vi "Choreo_SwerveSample_Unpack.vi"(9 "StartByte":i32, 11 "RawData":u8[](array[numeric])) -> (1 "NextByte":i32, 3 "ChoreoSwerveSample":T1)   [LabVIEW 2019, in "ChoreoLib.lvlib"]
doc: "Unpack a binary byte stream into a Swerve Trajectory Sample.\n\nInputs:\n -- RawData - Byte Array - Input byte stream\n -- StartByte - Integer - Starting byte (0 relative) to parse\n\nOutputsL:\n -- ChoreoSwerveSample - cluster - Swerve trajectory sample data\n -- NextByte - integer - Index into next byte to parse"
uses:
  ChoreoLib.lvlib
  TypeDef/ChoreoSwerveSample.ctl
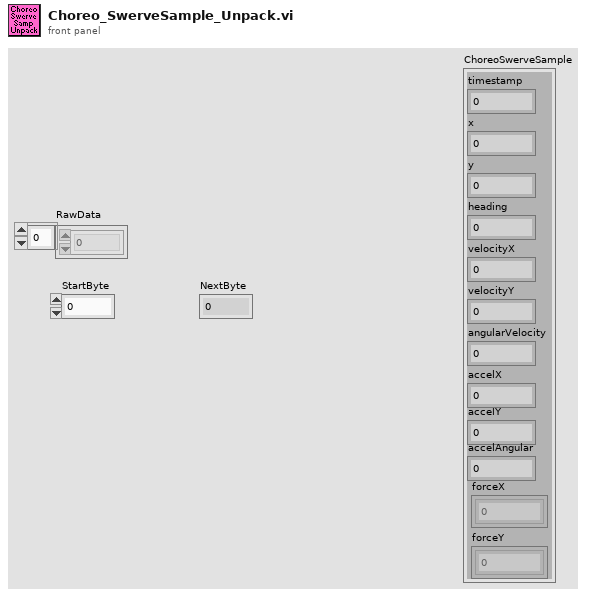
[diagram p1: front panel]
types:
  T1 = typedef "ChoreoLib.lvlib/ChoreoSwerveSample.ctl" = cluster{"timestamp":dbl, "x":dbl, "y":dbl, "heading":dbl, "velocityX":dbl, "velocityY":dbl, "angularVelocity":dbl, "accelX":dbl, "accelY":dbl, "accelAngular":dbl, "forceX":dbl[], "forceY":dbl[]}
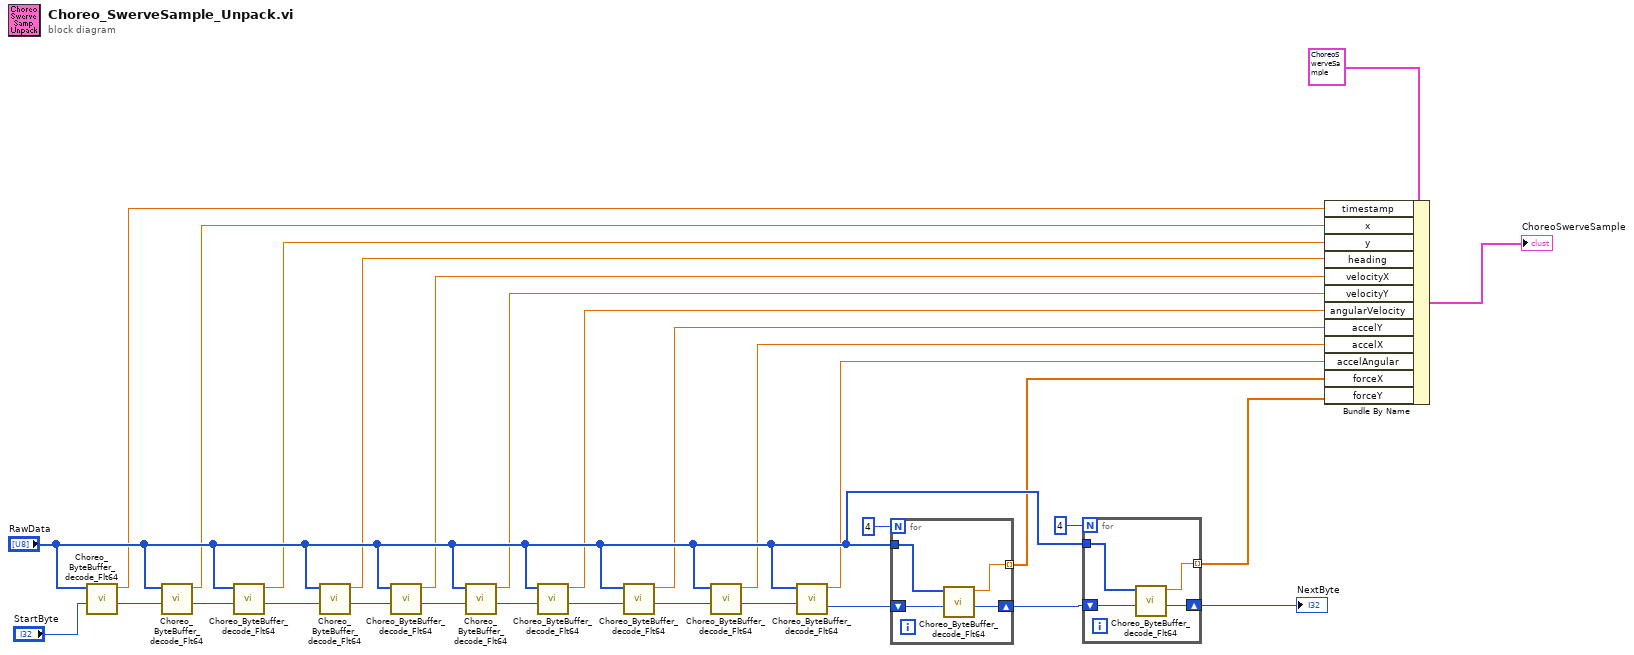
[diagram p0: block diagram]
diagram:
  n1 = call "Choreo_ByteBuffer_decode_Flt64.vi"("StartByte"="StartByte", "RawData"="RawData") -> ("NextByte"=w27:i32, "Flt64_Value"=w7:dbl)  [unwired: 8 in]
  n2 = call "Choreo_ByteBuffer_decode_Flt64.vi"("StartByte"=w27, "RawData"="RawData") -> ("NextByte"=w26:i32, "Flt64_Value"=w6:dbl)  [unwired: 8 in]
  n3 = call "Choreo_ByteBuffer_decode_Flt64.vi"("StartByte"=w26, "RawData"="RawData") -> ("NextByte"=w25:i32, "Flt64_Value"=w5:dbl)  [unwired: 8 in]
  n4 = call "Choreo_ByteBuffer_decode_Flt64.vi"("StartByte"=w25, "RawData"="RawData") -> ("NextByte"=w24:i32, "Flt64_Value"=w4:dbl)  [unwired: 8 in]
  n5 = call "Choreo_ByteBuffer_decode_Flt64.vi"("StartByte"=w24, "RawData"="RawData") -> ("NextByte"=w23:i32, "Flt64_Value"=w3:dbl)  [unwired: 8 in]
  n6 = call "Choreo_ByteBuffer_decode_Flt64.vi"("StartByte"=w23, "RawData"="RawData") -> ("NextByte"=w22:i32, "Flt64_Value"=w2:dbl)  [unwired: 8 in]
  n7 = call "Choreo_ByteBuffer_decode_Flt64.vi"("StartByte"=w22, "RawData"="RawData") -> ("NextByte"=w21:i32, "Flt64_Value"=w8:dbl)  [unwired: 8 in]
  n8 = call "Choreo_ByteBuffer_decode_Flt64.vi"("StartByte"=w21, "RawData"="RawData") -> ("NextByte"=w20:i32, "Flt64_Value"=w9:dbl)  [unwired: 8 in]
  n9 = call "Choreo_ByteBuffer_decode_Flt64.vi"("StartByte"=w20, "RawData"="RawData") -> ("NextByte"=w19:i32, "Flt64_Value"=w10:dbl)  [unwired: 8 in]
  n10 = call "Choreo_ByteBuffer_decode_Flt64.vi"("StartByte"=w19, "RawData"="RawData") -> ("NextByte"=w17:i32, "Flt64_Value"=w11:dbl)  [unwired: 8 in]
  n11 = for {
    N: 4 -> [_]
    tunnel: "RawData" -> [w34]
    shift-right: [w32] -> w14
    shift-left: w17 -> [w33]
    tunnel: [w31] -> w12 mode=indexing
    n12 = call "Choreo_ByteBuffer_decode_Flt64.vi"("StartByte"=w33, "RawData"=w34) -> ("NextByte"=w32:i32, "Flt64_Value"=w31:dbl)  [unwired: 8 in]
  }
  n13 = for {
    N: 4 -> [_]
    tunnel: "RawData" -> [w38]
    shift-right: [w36] -> w1
    shift-left: w14 -> [w37]
    tunnel: [w35] -> w13 mode=indexing
    n14 = call "Choreo_ByteBuffer_decode_Flt64.vi"("StartByte"=w37, "RawData"=w38) -> ("NextByte"=w36:i32, "Flt64_Value"=w35:dbl)  [unwired: 8 in]
  }
  "NextByte" <- w1
  n15 = Bundle By Name(cluster=T1 {"timestamp"=0.0, "x"=0.0, "y"=0.0, "heading"=0.0, "velocityX"=0.0, "velocityY"=0.0, "angularVelocity"=0.0, "accelX"=0.0, "accelY"=0.0, "accelAngular"=0.0, "forceX"=[], "forceY"=[]} ("ChoreoSwerveSample 2"), "timestamp"=w7, "x"=w6, "y"=w5, "heading"=w4, "velocityX"=w3, "velocityY"=w2, "angularVelocity"=w8, "accelY"=w9, "accelX"=w10, "accelAngular"=w11, "forceX"=w12, "forceY"=w13) -> (→"ChoreoSwerveSample":T1)
